vi "Test Load Snapshot - probes.vi"() -> (0 "error out":errorcluster)   [LabVIEW 2020]
doc: "Test loading snapshot with only probes."
uses:
  <vilib>/addons/_JKI Toolkits/Caraya/classes/Test/Test.lvclass
  src/Public API.lvlib
  src/Path Getter Mock/Path Getter Mock.lvclass
  src/Type Definitions/Snapshot Handling Options--cluster.ctl
  src/Type Definitions/Class Name--enum.ctl
  <vilib>/Utility/miscctls.llb/LVBreakpointStatusEnum.ctl
  src/Type Definitions/Breakpoint--cluster.ctl
  src/Type Definitions/Debug Snapshot--cluster.ctl
  C:/Users/juanj/Documents/hasbun_wood_engineering/github/Debug-Snapshots-for-LabVIEW/src/Path Getter Mock/Path Getter Mock.lvclass
  C:/Users/juanj/Documents/hasbun_wood_engineering/github/Debug-Snapshots-for-LabVIEW/src/IPath Getter/IPath Getter.lvclass
  <vilib>/addons/_JKI Toolkits/Caraya/classes/Assert/Assert.lvclass
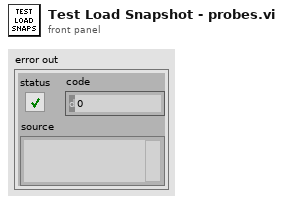
[diagram p1: front panel]
types:
  T1 = typedef "Breakpoint--cluster.ctl" = cluster{"UID":i32, "BP Status":T2, "Class Name":T3}
  T2 = typedef "LVBreakpointStatusEnum.ctl" = enum8{"Cleared Break", "Enabled Break", "Disabled Break"}
  T3 = typedef "Class Name--enum.ctl" = enum16{"Node", "Wire"}
  T4 = typedef "Debug Snapshot--cluster.ctl" = cluster{"VI Name":string, "Breakpoints":T1[], "Probes":i32[]}
  T5 = typedef "Snapshot Handling Options--cluster.ctl" = cluster{"Breakpoints":bool, "Probes":bool}
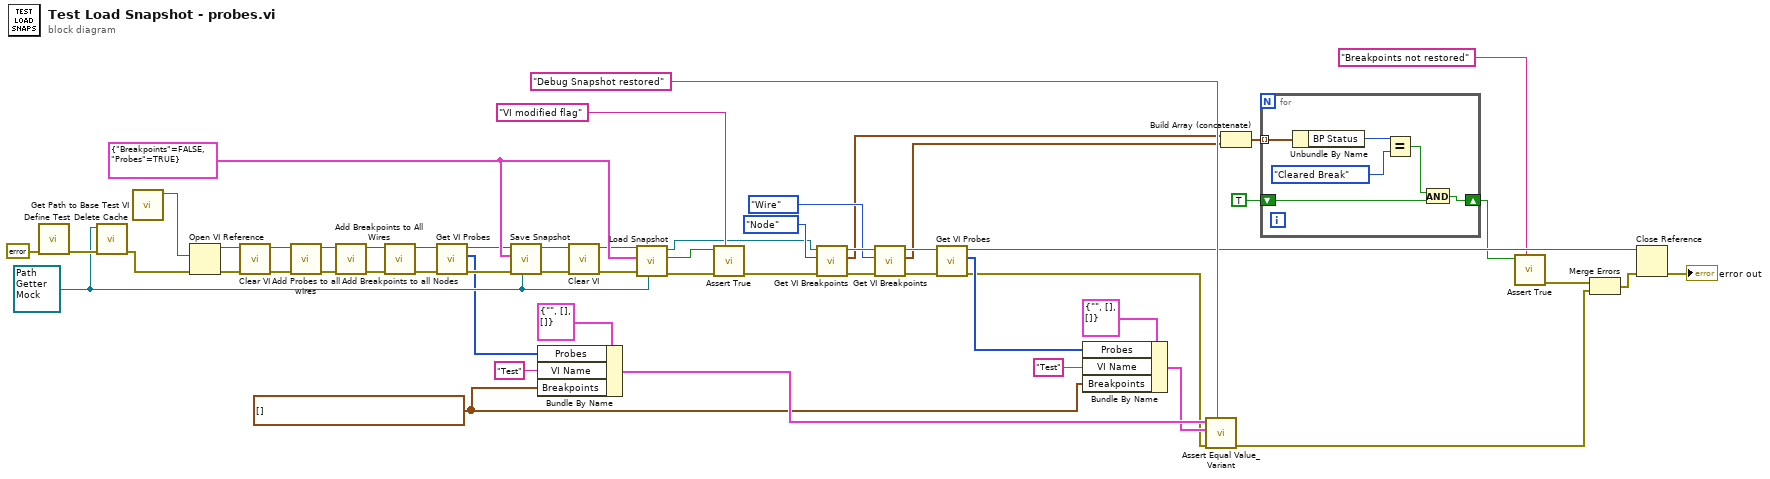
[diagram p0: block diagram]
diagram:
  w15 = T1[] [] ("Breakpoints")
  w43 = T5 {"Breakpoints"=FALSE, "Probes"=TRUE} ("Debug Elements Options")
  w19 = refnum<class "Path Getter Mock.lvclass"> refnum ("Path Getter Mock.lvclass")
  n1 = call <vilib>:"Define Test.vi"("error in (no error)"=errorcluster {"status"=FALSE, "code"=0, "source"=""}) -> ("error out"=w53:errorcluster)  [unwired: 9 in, 1 out]
  n2 = call "Delete Cache.vi"("error in"=w53, "IPath Getter.lvclass"=w19) -> ("error out"=w50:errorcluster)  [unwired: 9 in]
  n3 = call "Get Path to Base Test VI.vi"() -> ("Path"=w51:path)  [unwired: 11 in]
  n4 = Open VI Reference(vi path=w51, error in (no error)=w50) -> (vi reference=w4:refnum<vi>, error out=w52:errorcluster)  [unwired: 4 in]
  n5 = call "Clear VI.vi"("error in"=w52, "VI Refnum In"=w4) -> ("error out"=w5:errorcluster, "VI Refnum Out"=w3:refnum<vi>)  [unwired: 8 in]
  n6 = call "Add Probes to all wires.vi"("error in"=w5, "VI Refnum In"=w3) -> ("error out"=w48:errorcluster, "VI Refnum Out"=w49:refnum<vi>)  [unwired: 8 in]
  n7 = call "Add Breakpoints to All Wires.vi"("error in"=w48, "VI Refnum In"=w49) -> ("error out"=w46:errorcluster, "VI Refnum Out"=w47:refnum<vi>)  [unwired: 8 in]
  n8 = call "Add Breakpoints to all Nodes.vi"("error in"=w46, "VI Refnum In"=w47) -> ("error out"=w41:errorcluster, "VI Refnum Out"=w42:refnum<vi>)  [unwired: 8 in]
  n9 = call "Get VI Probes.vi"("error in"=w41, "VI Reference in"=w42) -> ("error out"=w17:errorcluster, "Probes"=w16:i32[], "VI Reference out"=w18:refnum<vi>)  [unwired: 7 in]
  n10 = call "Save Snapshot.vi"("IPath Getter in"=w19, "error in"=w17, "Debug Elements Options"=w43, "VI Reference in"=w18) -> ("error out"=w45:errorcluster, "VI Reference out"=w2:refnum<vi>)  [unwired: 6 in]
  n11 = Bundle By Name(cluster=T4 {"VI Name"="", "Breakpoints"=[], "Probes"=[]} ("Debug Snapshot"), "Probes"=w16, "VI Name"="Test", "Breakpoints"=w15) -> (w24:T4)
  n12 = call "Clear VI.vi"("error in"=w45, "VI Refnum In"=w2) -> ("error out"=w44:errorcluster, "VI Refnum Out"=w1:refnum<vi>)  [unwired: 8 in]
  n13 = call "Load Snapshot.vi"("IPath Getter in"=w19, "error in"=w44, "Debug Elements Options"=w43, "VI Reference in"=w1) -> ("error out"=w31:errorcluster, "VI Modified"=w32:bool, "VI Reference out"=w29:refnum<vi>)  [unwired: 5 in]
  n14 = call <vilib>:"Assert True.vi"("Label"="VI modified flag", "error in (no error)"=w31, "True?"=w32) -> ("error out"=w28:errorcluster)  [unwired: 7 in, 1 out]
  n15 = call "Get VI Breakpoints.vi"("error in"=w28, "Class Name"=Class_Name--enum."Node", "VI Reference in"=w29) -> ("error out"=w37:errorcluster, "Breakpoints"=w14:T1[], "VI Reference out"=w38:refnum<vi>)  [unwired: 6 in]
  n16 = call "Get VI Breakpoints.vi"("error in"=w37, "Class Name"=Class_Name--enum."Wire", "VI Reference in"=w38) -> ("error out"=w35:errorcluster, "Breakpoints"=w13:T1[], "VI Reference out"=w36:refnum<vi>)  [unwired: 6 in]
  n17 = call "Get VI Probes.vi"("error in"=w35, "VI Reference in"=w36) -> ("error out"=w21:errorcluster, "Probes"=w25:i32[], "VI Reference out"=w20:refnum<vi>)  [unwired: 7 in]
  n18 = Bundle By Name(cluster=T4 {"VI Name"="", "Breakpoints"=[], "Probes"=[]} ("Debug Snapshot"), "Probes"=w25, "VI Name"="Test", "Breakpoints"=w15) -> (w23:T4)
  n19 = call <vilib>:"Assert Equal Value_Variant.vi"("Label"="Debug Snapshot restored", "error in (no error)"=w21, "Actual"=w23, "Expected"=w24) -> ("error out"=w9:errorcluster)  [unwired: 6 in, 1 out]
  n20 = Build Array (concatenate)(w14, w13) -> (w12:T1[])
  n21 = for {
    tunnel: w12 -> [w61] mode=indexing
    shift-right: [w56] -> w7
    shift-left: TRUE -> [w57]
    n22 = Unbundle By Name(w61) -> ("BP Status"=w60:T2)
    n23 = Equal?(x=w60, y=LVBreakpointStatusEnum."Cleared Break") -> (x = y?=w58:bool)
    n24 = And(x=w58, y=w57) -> (x .and. y?=w56:bool)
  }
  n25 = call <vilib>:"Assert True.vi"("Label"="Breakpoints not restored", "True?"=w7) -> ("error out"=w10:errorcluster)  [unwired: 8 in, 1 out]
  n26 = Merge Errors(w10, w9) -> (w8:errorcluster)
  n27 = Close Reference(reference=w20, error in (no error)=w8) -> (error out=→"error out":errorcluster)
